vi "Parameter Setup.vi"() -> (0 "Serial Numbers":string[](array[string]), 1 "Slewtime (out)":u16(ring) items=["1", ".1", "10"], 2 "Gatetime(out)":string, 3 "Number of Units(out)":i32 min=1 max=32 step=1, 4 "Soak Time(out)":u16(ring) items=["10", "5", "15", "30", "60", "90", "120"], 5 "Channel(s) (out)":u16(ring) items=["1+2", "1", "2", "3"], 6 "Temp Type(out)":i32=2 min=2 max=15, 8 "Unit_Number(out)":string="XXXXXXXXXXX", 9 "Work Order(out)":string="XXXXX-XXX")   [LabVIEW 2024]
panel:
  in  "Channel(s)":u16(ring) items=["1+2", "1", "2", "3"]
  in  "Soak Time":u16(ring) items=["10", "5", "0", "15", "30", "60", "90", "120"]
  in  "Slew Rate":u16(ring) items=["2", "1", "0.5"]
  in  "Gatetime":u16(ring) items=["1", ".1", "10"]
  in  "Unit_Number":string
  in  "Work Order":string
  in  "Temp Type":i32=1 min=1 max=20 step=1
  in  "Enter":bool
  in  "Number of Units":i32=1 min=1 max=32 step=1
  # "Please Enter Values \nFor Each Text Box"
  # "Temp Type Guide:\n1: -40C to 85C @ 5C steps\n2: -20C to 85C @ 5C steps\n3: -20C to 70C @ 5C steps\n4: -40C to 85C @ 10C steps\n5: -20C to 85C @ 10C steps\n6: -20C to 70C @ 10C steps\n7: 0C to 50C @ 5C steps\n8: -20C to 85C @ 20C steps\n9: -40C to 85C @ 20C steps\n10: -40C to 70C @ 5C steps\n11: -25C to 75C @ 5C steps\n12: 85C,75C,70C,55C,40C,25C,10C,0C,-20C,-35C,-40C\n13: 75C,70C,55C,40C,25C,10C,0C,-20C,-35C,-40C\n14: 60C,40C,25C,10C,0C,-10C\n15-20: Custom"
  # "Legend:\nSlew Rate: # of Degrees changed \nper minute\nSoak Time: Amount of time soaked\nat each temperature step\nChannel(s): Channels used on\nFrequency Counter (1+2 = 16 and 16)"
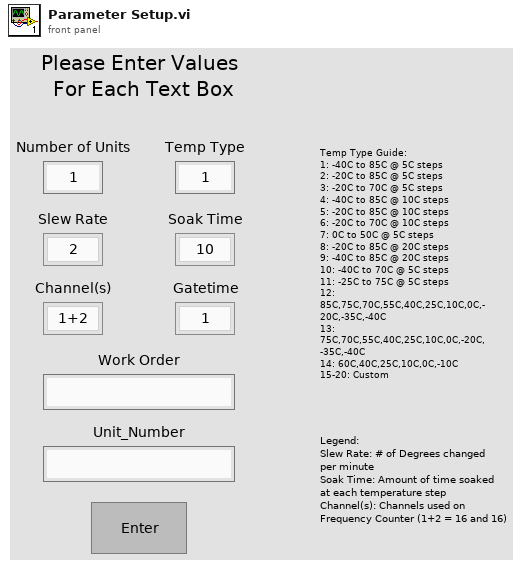
[diagram p1: front panel]
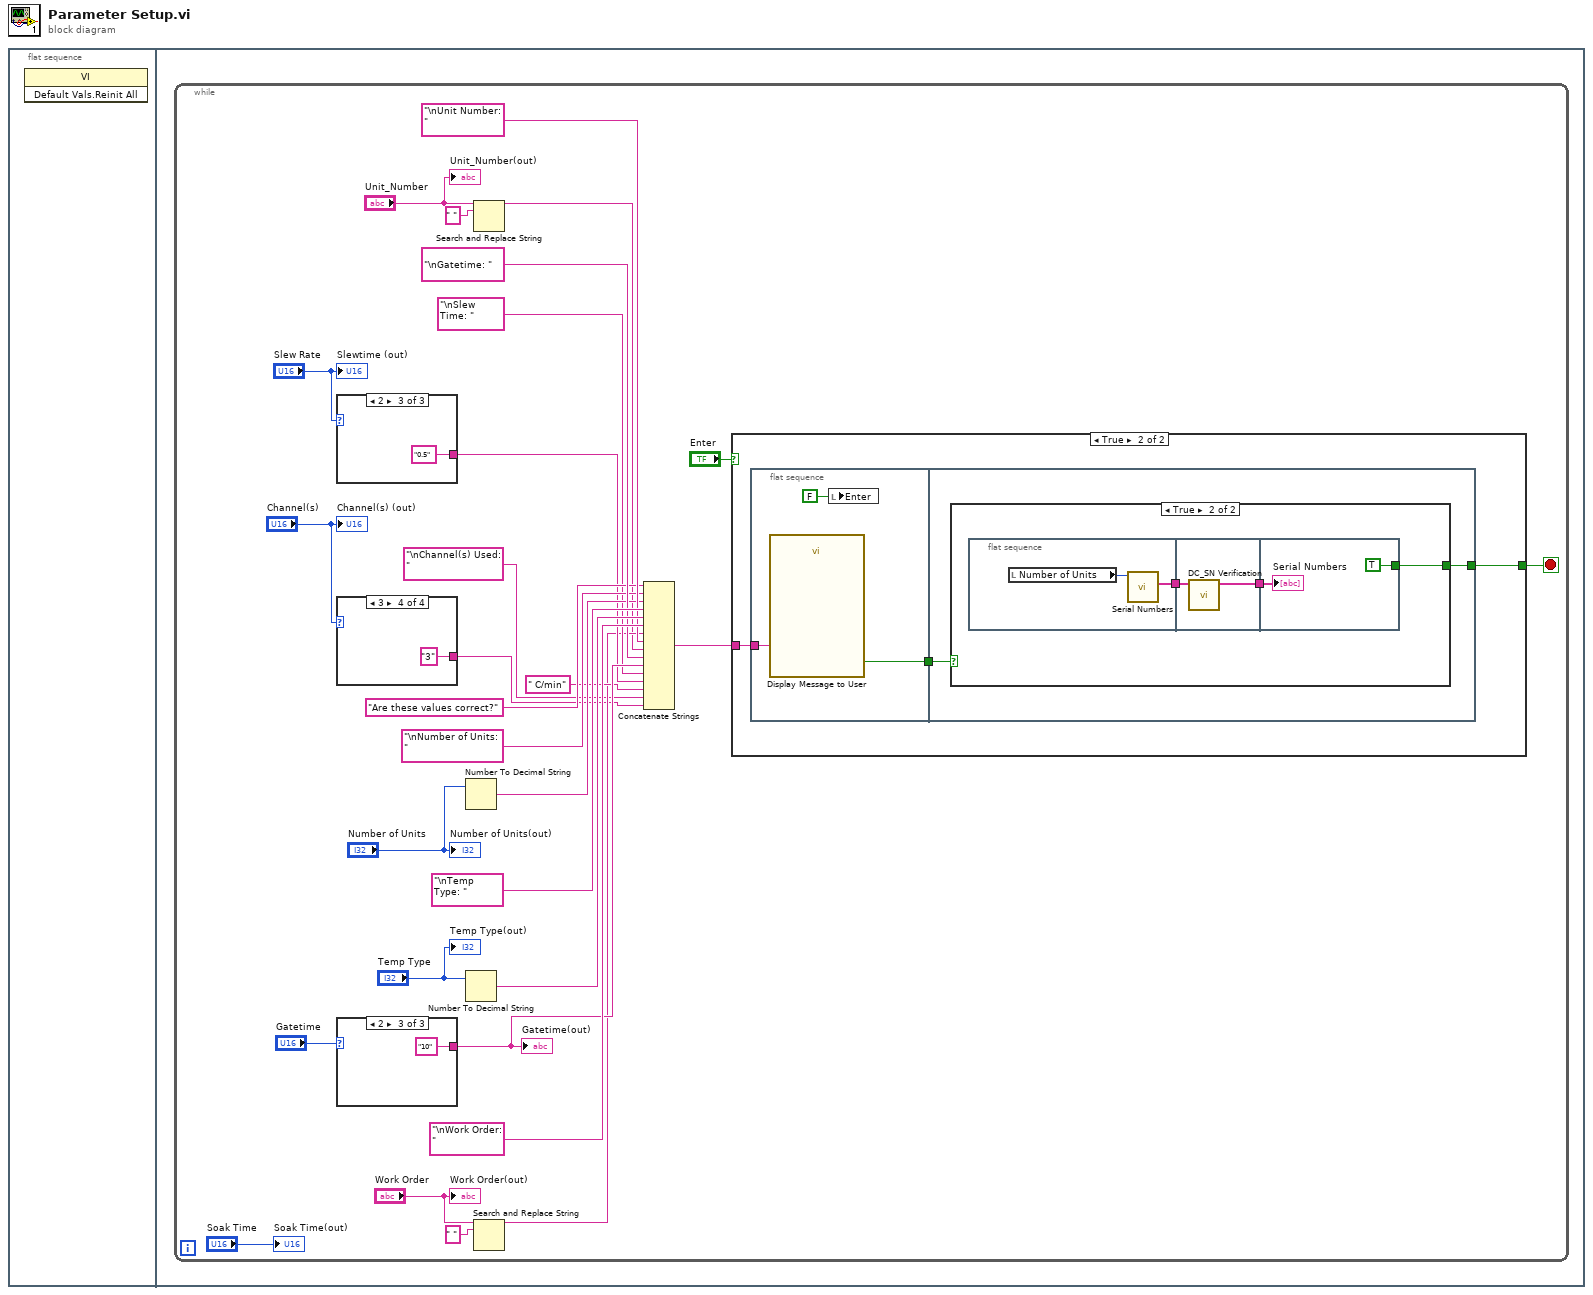
[diagram p0: block diagram]
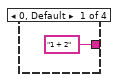
[diagram p2: hidden frame]
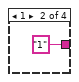
[diagram p3: hidden frame]
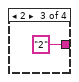
[diagram p4: hidden frame]
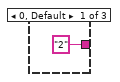
[diagram p5: hidden frame]
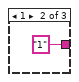
[diagram p6: hidden frame]
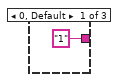
[diagram p7: hidden frame]
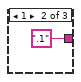
[diagram p8: hidden frame]
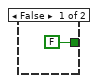
[diagram p9: hidden frame]
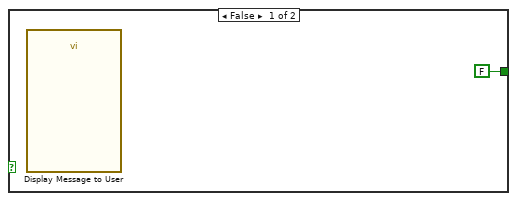
[diagram p10: hidden frame]
diagram:
  n1 = flat-sequence {
    frame #0 {
      n2 = invoke class="VI" method="Default Vals.Reinit All"() -> ()  [unwired: 3 in, 3 out]
    }
    frame #1 {
      n3 = while {
        stop <- w28 stop-if-true
        n4 = case shown="2" "Slew Rate" {
          tunnel: ["2" "1" "0.5"] -> w11
          frame 0, Default {
          }
          frame 1 {
          }
          frame 2 {
          }
        }
        n5 = case shown="3" "Channel(s)" {
          tunnel: ["1 + 2" "1" "2" "3"] -> w1
          frame 0, Default {
          }
          frame 1 {
          }
          frame 2 {
          }
          frame 3 {
          }
        }
        n6 = case shown="2" "Gatetime" {
          tunnel: ["1" ".1" "10"] -> w18
          frame 0, Default {
          }
          frame 1 {
          }
          frame 2 {
          }
        }
        "Gatetime(out)" <- w18
        n7 = Number To Decimal String(number="Number of Units") -> (decimal integer string=w17:string)  [unwired: 1 in]
        n8 = Number To Decimal String(number="Temp Type") -> (decimal integer string=w23:string)  [unwired: 1 in]
        n9 = Search and Replace String(input string="Unit_Number", search string=" ") -> (result string=w4:string)  [unwired: 6 in, 3 out]
        n10 = Search and Replace String(input string="Work Order", search string=" ") -> (result string=w7:string)  [unwired: 6 in, 3 out]
        n11 = Concatenate Strings("Are these values correct?", "\nNumber of Units: " ("string"), w17, "\nTemp Type: " ("string"), w23, "\nWork Order: " ("string"), w7, "\nUnit Number: " ("string"), w4, "\nGatetime: " ("string"), w18, "\nSlew Time: " ("string"), w11, " C/min" ("string"), "\nChannel(s) Used: " ("string"), w1) -> (w26:string)
        n12 = case shown="True" "Enter" {
          tunnel: [FALSE w43] -> w28
          tunnel: w26 -> [_ w41]
          frame False {
          }
          frame True {
            n13 = flat-sequence {
              tunnel: [w46] -> w42
              tunnel: w41 -> [w44]
              tunnel: [w48] -> w43
              tunnel: w42 -> [w47]
              frame #0 {
                n14 = call "Display Message to User"("Message"=w44) -> ("Yes"=w46:bool)  [unwired: 9 in, 1 out]
                n15 = local write "Enter"(FALSE ("Enter")) -> ()
              }
              frame #1 {
                n16 = case shown="True" w47 {
                  tunnel: [FALSE w52] -> w48
                  frame False {
                    n17 = call "Display Message to User"() -> ()  [unwired: 10 in, 2 out]
                  }
                  frame True {
                    n18 = flat-sequence {
                      tunnel: [w53] -> w51
                      tunnel: w51 -> [w56]
                      tunnel: [w55] -> w50
                      tunnel: [TRUE] -> w52
                      tunnel: w50 -> [w57]
                      frame #0 {
                        n19 = local read "Number of Units"() -> (w54:i32)
                        n20 = call "Serial Numbers.vi"("Total Number of Units"=w54) -> ("Serial Numbers"=w53:string[])  [unwired: 10 in]
                      }
                      frame #1 {
                        n21 = call "DC_SN Verification.vi"("Serial Numbers"=w56) -> ("Serial Numbers(out)"=w55:string[])  [unwired: 10 in]
                      }
                      frame #2 {
                        "Serial Numbers" <- w57
                      }
                    }
                  }
                }
              }
            }
          }
        }
        "Number of Units(out)" <- "Number of Units"
        "Temp Type(out)" <- "Temp Type"
        "Work Order(out)" <- "Work Order"
        "Unit_Number(out)" <- "Unit_Number"
        "Slewtime (out)" <- "Slew Rate"
        "Soak Time(out)" <- "Soak Time"
        "Channel(s) (out)" <- "Channel(s)"
      }
    }
  }
